vi "Request Processing Loop to Refresh Tree.vi"(6 "Force Update":bool, 8 "error in (no error)":errorcluster, 10 "Queue in":refnum<queue>, 11 "ConfigInfo in":T1) -> (0 "error out":errorcluster)   [LabVIEW 2013, in "LVTM.lvlib"]
uses:
  LVTM.lvlib
  Controls_LVTM/LVTM_Config_Info.ctl
  Controls_LVTM/View.ctl
  Controls_LVTM/SharedDataDVR.ctl
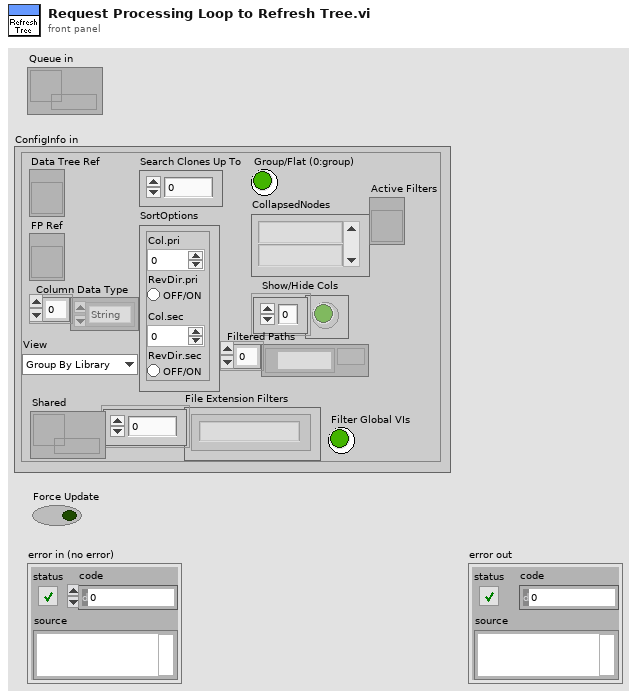
[diagram p1: front panel]
types:
  T1 = typedef "LVTM.lvlib/LVTM_Config_Info.ctl" = cluster{"Data Tree Ref":refnum<vi>, "FP Ref":refnum<vi>, "Column Data Type":enum16{"String", "Numeric"}[], "Search Clones Up To":i32, "SortOptions":cluster{"Col.pri":i32, "RevDir.pri":bool, "Col.sec":i32, "RevDir.sec":bool}, "Group/Flat (0:group)":bool, "CollapsedNodes":string[], "Show/Hide Cols":bool[], "Filtered Paths":path[], "View":T2, "File Extension Filters":string[], "Filter Global VIs":bool, "Shared":refnum<data-value>, "Active Filters":refnum<vi>}
  T2 = typedef "LVTM.lvlib/View.ctl" = enum16{"Group By Library", "Group By Folder", "Flat List"}
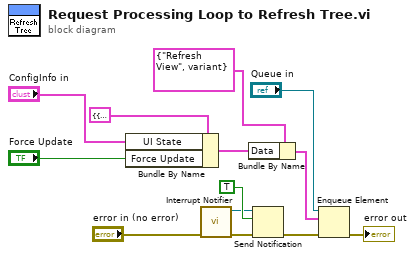
[diagram p0: block diagram]
diagram:
  n1 = Bundle By Name(cluster=cluster{"UI State":T1, "Force Update":bool} {"UI State"={"Data Tree Ref"=refnum, "FP Ref"=refnum, "Column Data Type"=[], "Search Clones Up To"=0, "SortOptions"={"Col.pri"=0, "RevDir.pri"=FALSE, "Col.sec"=0, "RevDir.sec"=FALSE}, "Group/Flat (0:group)"=FALSE, "CollapsedNodes"=[], "Show/Hide Cols"=[], "Filtered Paths"=[], "View"=enum."Group By Library", "File Extension Filters"=[], "Filter Global VIs"=FALSE, "Shared"=refnum, "Active Filters"=refnum}, "Force Update"=FALSE}, "UI State"="ConfigInfo in", "Force Update"="Force Update") -> (w5:cluster{"UI State":T1, "Force Update":bool})
  n2 = call "Interrupt Notifier.vi"("error in"="error in (no error)") -> ("error out"=w11:errorcluster, "Notifier out"=w10:refnum<notifier>)  [unwired: 9 in]
  n3 = Bundle By Name(cluster=cluster{"Command":string, "Data":variant} {"Command"="Refresh View", "Data"=variant} ("element"), "Data"=w5) -> (w3:cluster{"Command":string, "Data":variant})
  n4 = Send Notification(notification=TRUE, notifier=w10, error in (no error)=w11) -> (error out=w13:errorcluster)  [unwired: 1 out]
  n5 = Enqueue Element(queue="Queue in", element=w3, error in (no error)=w13) -> (error out=→"error out":errorcluster)  [unwired: 1 in, 2 out]
